vi "Get UI Details.vi"() -> ()   [LabVIEW 2020, in "NIDCPowerSourceDCVoltage.lvlib"]
uses:
  NIDCPowerSourceDCVoltage.lvlib
  <vilib>/MeasurementLink/MeasurementLink Measurement Server/Helpers/TypeDefs/User Interface Information.ctl
  <vilib>/MeasurementLink/MeasurementLink Measurement Server/MeasurementLink Measurement Server.lvlib
panel:
  out "error out":errorcluster
  in  "error in (no error)":errorcluster
  out "user interface details":T1[](array[typedef])
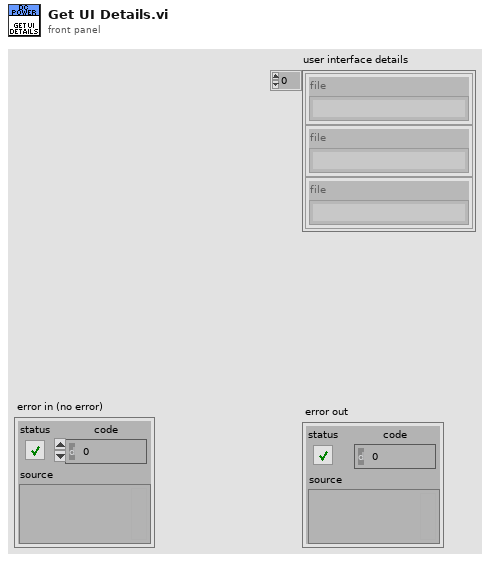
[diagram p1: front panel]
types:
  T1 = typedef "MeasurementLink Measurement Server.lvlib/User Interface Information.ctl" = cluster{"file":string}
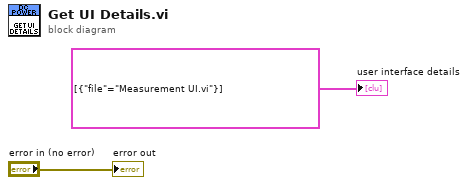
[diagram p0: block diagram]
diagram:
  "user interface details" <- T1[] [{"file"="Measurement UI.vi"}] ("appended array")
  "error out" <- "error in (no error)"
